vi "mod_LDPC Calculate Likelihoods (BSC).vi"(0 "bitstream in":i8[](array[numeric]), 5 "Noise (bit flip probability)":dbl=0.0001, 11 "error in (no error)":errorcluster) -> (4 "likelihoods out":dbl[](array[numeric]), 15 "error out":errorcluster)   [LabVIEW 2020, in "niDMT.lvlib"]
uses:
  <vilib>/addons/Modulation/niDMT.lvlib
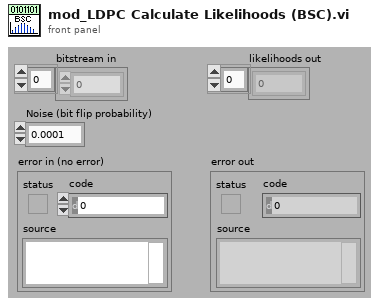
[diagram p1: front panel]
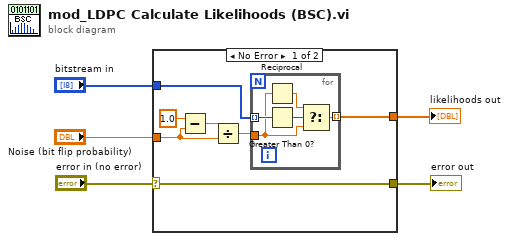
[diagram p0: block diagram]
diagram:
  n1 = case shown="No Error" "error in (no error)" {
    selector: "error in (no error)" -> [w6 w18]
    tunnel: "Noise (bit flip probability)" -> [w9 _]
    tunnel: "bitstream in" -> [w8 _]
    tunnel: [w7 _] -> w3
    tunnel: [w6 w18] -> w1
    frame No Error {
      n2 = Subtract(x=1.0, y=w9) -> (x-y=w10:dbl)
      n3 = Divide(x=w10, y=w9) -> (x/y=w12:dbl)
      n4 = for {
        tunnel: w8 -> [w17] mode=indexing
        tunnel: w12 -> [w13]
        tunnel: [w15] -> w7 mode=indexing
        n5 = Reciprocal(x=w13) -> (1/x=w14:dbl)
        n6 = Greater Than 0?(x=w17) -> (x > 0?=w16:bool)
        n7 = Select(t=w14, s=w16, f=w13) -> (s? t:f=w15:dbl)
      }
    }
    frame Error {
    }
  }
  "likelihoods out" <- w3
  "error out" <- w1
